vi "get_street_names.vi"(11 "Strassen in":T1[](array[typedef])) -> (3 "streets":string[](array[string]))   [LabVIEW 2019]
uses:
  Strasse.ctl
  Verbindung.ctl
  Strassentyp.ctl
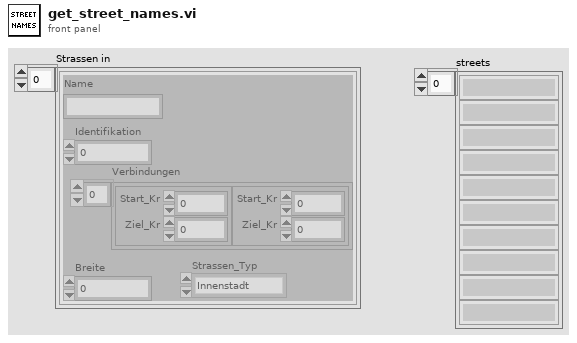
[diagram p1: front panel]
types:
  T1 = typedef "Strasse.ctl" = cluster{"Name":string, "Identifikation":u8, "Verbindungen":T2[], "Breite":u8, "Strassen_Typ":T3}
  T2 = typedef "Verbindung.ctl" = cluster{"Start_Kr":u16, "Ziel_Kr":u16}
  T3 = typedef "Strassentyp.ctl" = enum16{"Innenstadt", "Stadt", "Land"}
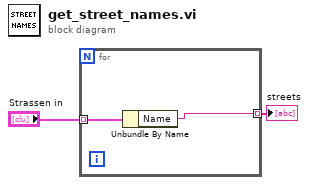
[diagram p0: block diagram]
diagram:
  n1 = for {
    tunnel: "Strassen in" -> [w4] mode=indexing
    tunnel: [w3] -> w1 mode=indexing
    n2 = Unbundle By Name(w4) -> ("Name"=w3:string)
  }
  "streets" <- w1
